vi "LCDDrawPixel.vi"(7 "pixelState":i32(ring) items=["PIXEL_STATE_OFF", "PIXEL_STATE_ON", "PIXEL_STATE_INVERT"], 8 "error in (no error)":errorcluster, 9 "y":i32, 10 "x":i32, 11 "Device In":u64) -> (0 "error out":errorcluster, 3 "Device Out":u64)   [LabVIEW 2012, in "Phidget LCD.lvlib"]
doc: "${DrawPixel:Header}"
uses:
  <instrlib>/Phidgets/Phidget LCD/Phidget LCD.lvlib
  <instrlib>/Phidgets/Phidget Common/Phidget Common.lvlib
  phidget22.dll
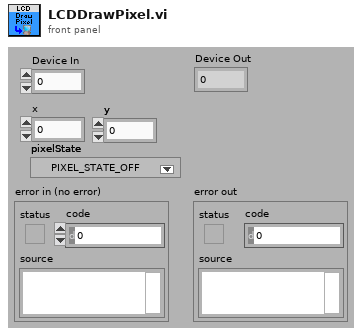
[diagram p1: front panel]
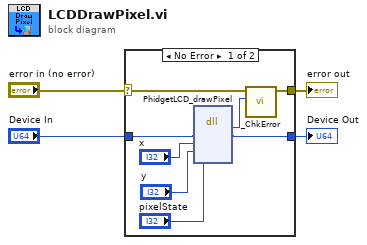
[diagram p0: block diagram]
diagram:
  n1 = case shown="No Error" "error in (no error)" {
    selector: "error in (no error)" -> [w12 w14]
    tunnel: [w11 w14] -> w3
    tunnel: "Device In" -> [w10 w13]
    tunnel: [w9 w13] -> w1
    frame No Error {
      n2 = dll-call lib="phidget22.*" fn="PhidgetLCD_drawPixel"("phid"=w10, "x"="x", "y"="y", "state"="pixelState") -> ("return type"=w8:i32, "phid"=w9:u64)  [unwired: 6 in, 2 out]
      n3 = call <instrlib>:"_ChkError.vi"("Return Code"=w8, "error in (no error)"=w12) -> ("error out"=w11:errorcluster)  [unwired: 9 in]
    }
    frame Error {
    }
  }
  "error out" <- w3
  "Device Out" <- w1
